vi "Debug_Convert_Data_to_String.vi"(8 "error in (no error)":errorcluster, 11 "AB_EXE in":refnum<class "AB_EXE.lvclass">) -> (0 "error out":errorcluster, 2 "classData":string, 3 "AB_EXE out":refnum<class "AB_EXE.lvclass">)   [LabVIEW 2020, in "AB_EXE.lvclass"]
uses:
  <vilib>/AppBuilder/AB_Classes/EXE/AB_EXE.lvclass
  <vilib>/AppBuilder/AB_Classes/EXE/AB_EXE.lvclass/AB_EXE.ctl
  <vilib>/AppBuilder/AB_Classes/Application/AB_Application.lvclass
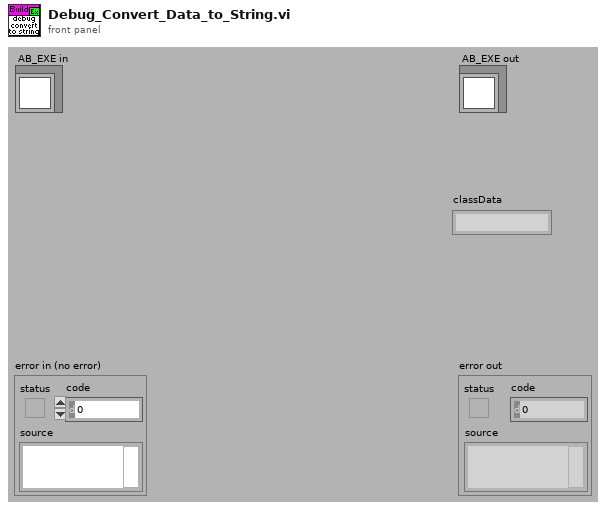
[diagram p1: front panel]
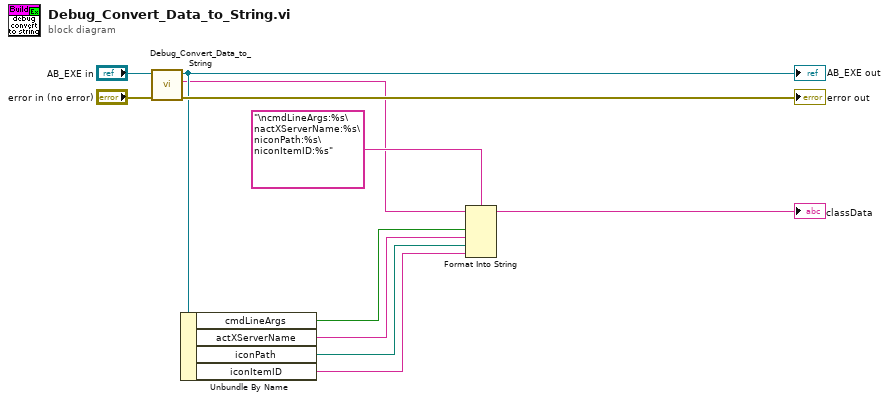
[diagram p0: block diagram]
diagram:
  n1 = call-parent "Debug_Convert_Data_to_String.vi"("error in (no error)"="error in (no error)", "AB_Application in"="AB_EXE in") -> ("error out"=→"error out":errorcluster, "classData"=w2:string, "AB_Application out"=w3:refnum<class "AB_EXE.lvclass">)  [unwired: 7 in]
  "AB_EXE out" <- w3
  n2 = Unbundle By Name(w3) -> ("cmdLineArgs"=w7:bool, "actXServerName"=w6:string, "iconPath"=w5:path, "iconItemID"=w4:string)
  n3 = Format Into String(format string="\ncmdLineArgs:%s\nactXServerName:%s\niconPath:%s\niconItemID:%s", initial string=w2, w7, w6, w5, w4) -> (resulting string=→"classData":string)  [unwired: 1 in, 1 out]
